vi "Init Hardware.vi"(8 "error in (no error)":errorcluster, 11 "Oxford PS Driver in":refnum<class "Oxford PS Driver.lvclass">) -> (0 "error out":errorcluster, 3 "Oxford PS Driver out":refnum<class "Oxford PS Driver.lvclass">)   [LabVIEW 2016, in "Oxford PS Driver.lvclass"]
uses:
  Oxford PS Driver.lvclass
  C:/github/NHMFL_Core/Libraries/Instruments/Instrument Driver/Instrument Driver.lvclass
  Instrument Driver/Instrument Driver.lvclass/Instrument Driver.ctl
  Instrument Driver/Read Recorder name.vi
  Instrument Driver/Write Channel names.vi
  Instrument Driver/Write Channel units.vi
  Simple VISA Reader/Simple VISA Reader Driver.lvclass
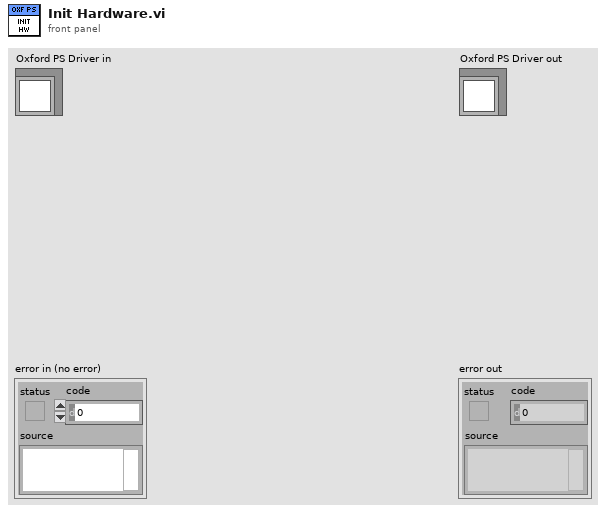
[diagram p1: front panel]
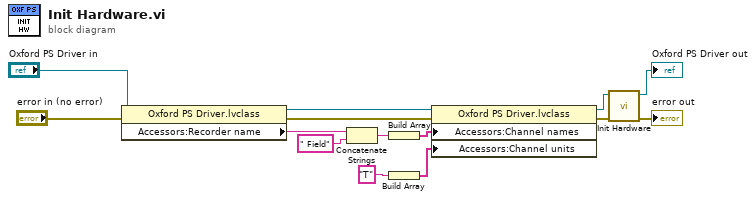
[diagram p0: block diagram]
diagram:
  n1 = property class="Oxford PS Driver.lvclass"(reference="Oxford PS Driver in", error in="error in (no error)") -> (reference out=w8:refnum<class "Oxford PS Driver.lvclass">, error out=w7:errorcluster, "Accessors:Recorder name"=w5:string)
  n2 = Concatenate Strings(w5, " Field") -> (w6:string)
  n3 = Build Array(w6) -> (w11:string[])
  n4 = Build Array("T") -> (w9:string[])
  n5 = property class="Oxford PS Driver.lvclass"(reference=w8, error in=w7, "Accessors:Channel names"=w11, "Accessors:Channel units"=w9) -> (reference out=w3:refnum<class "Oxford PS Driver.lvclass">, error out=w2:errorcluster)
  n6 = call-parent "Init Hardware.vi"("error in (no error)"=w2, "Instrument Driver in"=w3) -> ("error out"=→"error out":errorcluster, "Instrument Driver out"=→"Oxford PS Driver out":refnum<class "Oxford PS Driver.lvclass">)  [unwired: 8 in]
